vi "get Over Pressure Strategy.vi"(8 "error in (no error)":errorcluster, 10 "strategy":u32, 11 "pumpIndex":u32) -> (0 "error out":errorcluster, 2 "strategy out":u32, 3 "function return":i32)   [LabVIEW 2018, in "AsiaPumpInterface.lvlib"]
doc: "extern ASIAPUMP_INTERFACE_API BOOL getOverPressureStrategy( unsigned int pumpIndex ,\n unsigned int * strategy );"
uses:
  <userlib>/AsiaPumpInterface/AsiaPumpInterface.lvlib
  <userlib>/AsiaPumpInterface/AsiaPumpInterface.dll
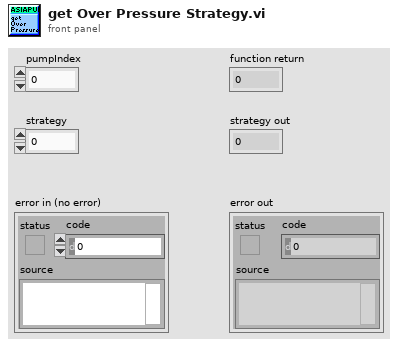
[diagram p1: front panel]
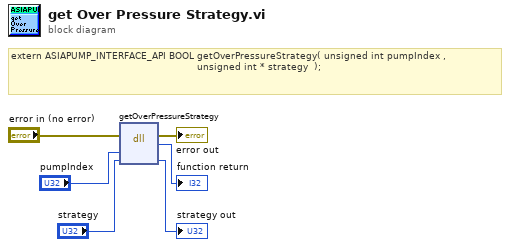
[diagram p0: block diagram]
diagram:
  # "extern ASIAPUMP_INTERFACE_API BOOL getOverPressureStrategy( unsigned int pumpIndex ,\n                                                              unsigned int * strategy  );"
  n1 = dll-call lib="C:/Program Files (x86)/National Instruments/LabVIEW 2018/user.lib/AsiaPumpInterface/AsiaPumpInterface.*" fn="getOverPressureStrategy"(error in="error in (no error)", "pumpIndex"="pumpIndex", "strategy"="strategy") -> (error out=→"error out":errorcluster, →"function return":i32, "strategy"=→"strategy out":u32)  [unwired: 3 in, 1 out]
